vi "DepthSense NewFrame Callback With Globals.vi"(4 "User Parameter":variant, 6 "Control Ref":refnum<k24>, 7 "Event Common Data":T1) -> ()   [LabVIEW 2011]
uses:
  C:/Users/Behavior Room/Desktop/Kinect Mouse/DepthSense/FunctionPointerProxy/FunctionPointerProxy/bin/Release/FunctionPointerProxy.dll
  FunctionPointerProxy/FunctionPointerProxy/bin/Release/FunctionPointerProxy.dll
  <vilib>/Utility/importsl/GetValueByPointer/datatype.ctl
  DepthSense Global Status.vi
  <vilib>/Utility/importsl/GetValueByPointer/GetValueByPointer.xnode
  <userlib>/libOptrima-2-3/libOptrima-2-3.lvlib
  Program Files (x86)/National Instruments/LabVIEW 2011/resource/lvimptsl.dll
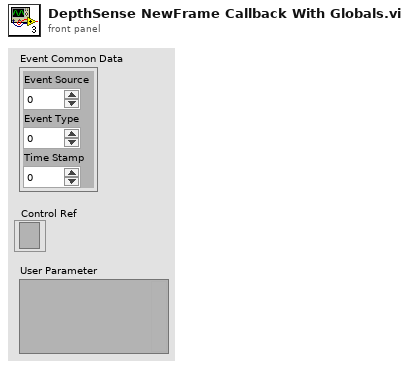
[diagram p1: front panel]
types:
  T1 = cluster{"Event Source":i32, "Event Type":u32, "Time Stamp":u32}
  T2 = typedef "Image Type" = u32
  T3 = cluster{"Camera Version":string, "Image Height":i32, "Image Width":i32, "Minimum Framerate":i32, "Maximum Framerate":i32, "Framerate":i32, "Close Mode":bool, "Denoising":bool, "Leakage Algorithm":bool, "Anti-Aliasing":bool, "Camera Status":i32, "API Version":string, "Light Intensity":i32, "Confidence Threshold":u16, "Range":sgl}
  T4 = typedef "IMAQ Image.ctl" = refnum<image>
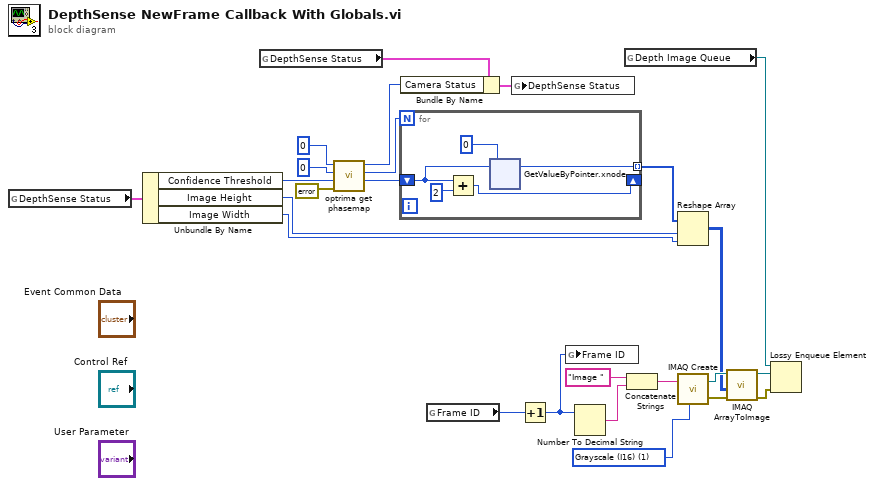
[diagram p0: block diagram]
diagram:
  w10 = T2 1 items=["Grayscale (U8)", "Grayscale (I16)", "Grayscale (SGL)", "Complex (CSG)", "RGB (U32)", "HSL (U32)", "RGB (U64)", "Grayscale (U16)"] ("Image Type")
  n1 = global read "DepthSense Global Status.vi" "DepthSense Status"() -> (w25:T3)
  n2 = Unbundle By Name(w25) -> ("Confidence Threshold"=w21:u16, "Image Height"=w16:i32, "Image Width"=w15:i32)
  n3 = global read "DepthSense Global Status.vi" "DepthSense Status"() -> (w23:T3)
  n4 = call <userlib>:"optrima get phasemap.vi"("error in (no error)"=errorcluster {"status"=FALSE, "code"=0, "source"=""}, "confidence_threshold"=w21, "length"=u32 0, "p_phase_map"=0) -> ("p_phase_map 2"=w1:i32, "length out"=w2:u32, "function return"=w22:i32)  [unwired: 4 in, 1 out]
  n5 = for {
    N: w2 -> [_]
    tunnel: [w26] -> w3 mode=indexing
    shift-right: [w28] -> _
    shift-left: w1 -> [w27]
    n6 = Add(x=w27, y=2) -> (x+y=w28:i32)
    n7 = xnode "GetValueByPointer.xnode"("Pointer"=w27, "InputType"=0 ("p_phase_map")) -> ("Output"=w26:i32)  [unwired: 2 in, 1 out]
  }
  n8 = Bundle By Name(cluster=w23, "Camera Status"=w22) -> (w24:T3)
  n9 = global read "DepthSense Global Status.vi" "Frame ID"() -> (w17:i32)
  n10 = global write "DepthSense Global Status.vi" "DepthSense Status"(w24) -> ()
  n11 = Increment(x=w17) -> (x+1=w14:i32)
  n12 = global write "DepthSense Global Status.vi" "Frame ID"(w14) -> ()
  n13 = Number To Decimal String(number=w14) -> (decimal integer string=w13:string)  [unwired: 1 in]
  n14 = global read "DepthSense Global Status.vi" "Depth Image Queue"() -> (w19:refnum<queue>)
  n15 = Concatenate Strings("Image " ("Image Name"), w13) -> (w11:string)
  n16 = Reshape Array(w3, w16, w15) -> (w5:i32[][])
  n17 = call "IMAQ Create"("Image Name"=w11, "Image Type"=w10) -> ("New Image"=w8:T4, "error out"=w9:errorcluster)  [unwired: 3 in]
  n18 = call "IMAQ ArrayToImage"("error in (no error)"=w9, "Image Pixels (I16)"=w5, "Image"=w8) -> ("error out"=w6:errorcluster, "Image Out"=w7:T4)  [unwired: 7 in]
  n19 = Lossy Enqueue Element(queue=w19, element=w7, error in (no error)=w6) -> ()  [unwired: 4 out]
